vi "SLL DE DAQ Engine Main.vi"(8 "error in (no error)":errorcluster) -> (0 "error out":errorcluster)   [LabVIEW 2013]
uses:
  Controls/SLL DE DAQ Parameters LV2Global Options.ctl
  Controls/SLL DE DAQ Global Options.ctl
  Controls/SLL DE DI Global Options.ctl
  Controls/SLL DE AI Global Options.ctl
  Controls/SLL DE DO Global Options.ctl
  Controls/SLL DE AO Global Options.ctl
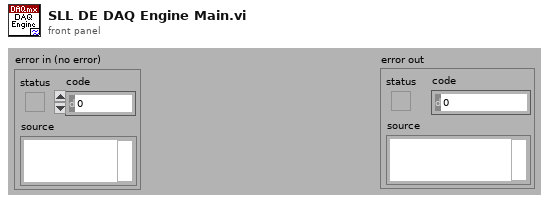
[diagram p1: front panel]
types:
  T1 = typedef "SLL DE DAQ Global Options.ctl" = enum16{"Init", "Write 1", "Read 1", "Write Array", "Read Array", "Clear"}
  T2 = typedef "SLL DE DAQ Parameters LV2Global Options.ctl" = enum16{"Read", "Write"}
  T3 = typedef "SLL DE DAQ Engine Parameters.ctl" = cluster{"Enable Engines":cluster{"AI Enable":bool, "AO Enable":bool, "DI Enable":bool, "DO Enable":bool}, "DAQ Control Type":cluster{"Analog Input":enum16{"Finite", "Continuous", "Driver"}, "Analog Output":enum16{"Finite", "Continuous", "Driver"}, "Digital Input":enum16{"Finite", "Continuous", "Driver"}, "Digital Output":enum16{"Finite", "Continuous", "Driver"}}, "DAQ Parameters":cluster{"AI Sampling Rate (Samples/Sec)":dbl, "MvgAVG Window Size (# of Points)":i32, "Enable Filter":bool, "Enable MvgAVG":bool, "Circular Buffer Size (Sec)":dbl, "AO Sampling Rate (Samples/Sec)":dbl, "Graph Update Rate (Samples/Sec)":dbl, "File Logging Rate (Samples/Sec)":i32}, "AO Safe Values":cluster{"Analog Outputs Name":T4, "Analog Outputs Safe Value":dbl}[], "DO Safe Values":cluster{"Digital Outputs Name":T5, "Digital Outputs Safe Value":bool}[], "DO Interconnected Lines":cluster{"First DO Line":string, "Second DO Line":string}[], "AI Channels Unit":cluster{"Channel Name":T6, "Channel Type":T7}[], "Units Information":cluster{"Channel Type":T7, "Unit Text":string, "Maximum":dbl, "Minmum":dbl, "Increments":dbl}[]}
  T4 = typedef "SLL DE List of Analog Outputs.ctl" = enum16{"None"}
  T5 = typedef "SLL DE List of Digital Outputs.ctl" = enum16{"STATION1_START TEST", "STATION1_STOP TEST", "STATION1_LIGHT1", "STATION1_LIGHT2", "STATION1_LIGHT3", "STATION1_SELECT_TEST", "STATION2_START TEST", "STATION2_STOP TEST", "STATION2_LIGHT1", "STATION2_LIGHT2", "STATION2_LIGHT3", "STATION2_SELECT_TEST", "STATION3_START TEST", "STATION3_STOP TEST", "STATION3_LIGHT1", "STATION3_LIGHT2", "STATION3_LIGHT3", "STATION3_SELECT_TEST", "STATION4_START TEST", "STATION4_STOP TEST", "STATION4_LIGHT1", "STATION4_LIGHT2", "STATION4_LIGHT3", "STATION4_SELECT_TEST"}
  T6 = typedef "SLL DE List of Analog Inputs.ctl" = enum16{"None"}
  T7 = typedef "SLL DE List of AI Channel Type.ctl" = enum16{"Pressure", "Flow", "Temperature", "Time Scale", "Voltage", "Current", "Frequency", "Sound", "Speed", "Torque", "Distance", "Channel Type 1", "Channel Type 2", "Channel Type 3"}
  T8 = typedef "SLL DE DI Global Options.ctl" = enum16{"Init", "Write Line", "Write Array", "Read Line", "Read Array", "Read Full Status", "Write Full Status"}
  T9 = typedef "SLL DE AO Global Options.ctl" = enum16{"Init", "Write Line", "Write Array", "Read Line", "Read Array", "Read Full Status", "Restart AO", "Send to Safe Mode", "Stop AO"}
  T10 = typedef "SLL DE DO Global Options.ctl" = enum16{"Init", "Write Line", "Write Array", "Write Full Status", "Read Line", "Read Array", "Read Full Status", "Restart DO", "Send to Safe Mode", "Stop DO"}
  T11 = typedef "SLL DE AI Global Options.ctl" = enum16{"Init", "Write Line", "Write Array", "Read Line", "Read Array", "Read Full Status", "Write Full Status"}
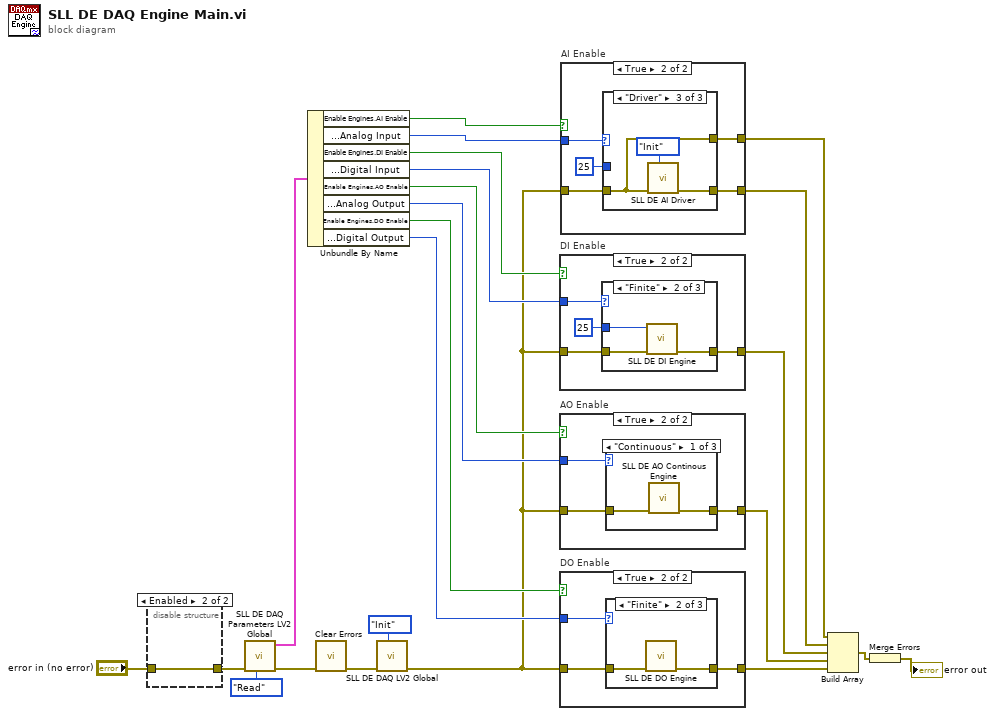
[diagram p0: block diagram]
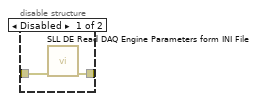
[diagram p2: hidden frame]
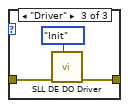
[diagram p5: hidden frame]
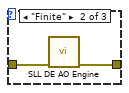
[diagram p7: hidden frame]
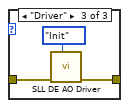
[diagram p8: hidden frame]
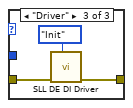
[diagram p11: hidden frame]
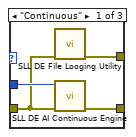
[diagram p13: hidden frame]
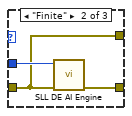
[diagram p14: hidden frame]
diagram:
  n1 = disable-structure shown="Enabled" {
    disable-tunnel: "error in (no error)" -> [w25 w26]
    disable-tunnel: [w24 w26] -> w9
    frame Disabled {
      n2 = call "SLL DE Read DAQ Engine Parameters form INI File.vi"("error in (no error)"=w25) -> ("error out"=w24:errorcluster)  [unwired: 10 out]
    }
    frame Enabled {
    }
  }
  n3 = call "SLL DE DAQ Parameters LV2 Global.vi"("Option"=SLL_DE_DAQ_Parameters_LV2Global_Options."Read", "Error in (no error)"=w9) -> ("Error out"=w8:errorcluster, "Global Info"=w7:T3)  [unwired: 1 in, 7 out]
  n4 = Unbundle By Name(w7) -> ("Enable Engines.AI Enable"=w4:bool, "DAQ Control Type.Analog Input"=w3:enum16{"Finite", "Continuous", "Driver"}, "Enable Engines.DI Enable"=w17:bool, "DAQ Control Type.Digital Input"=w18:enum16{"Finite", "Continuous", "Driver"}, "Enable Engines.AO Enable"=w15:bool, "DAQ Control Type.Analog Output"=w14:enum16{"Finite", "Continuous", "Driver"}, "Enable Engines.DO Enable"=w12:bool, "DAQ Control Type.Digital Output"=w11:enum16{"Finite", "Continuous", "Driver"})
  n5 = call <vilib>:"Clear Errors.vi"("error in (no error)"=w8) -> ("error out"=w6:errorcluster)  [unwired: 6 out]
  n6 = call "SLL DE DAQ LV2 Global.vi"("Option"=SLL_DE_DAQ_Global_Options."Init", "error in (no error)"=w6) -> ("error out"=w2:errorcluster)  [unwired: 4 in, 5 out]
  n7 = case "DI Enable" shown="True" w17 {
    tunnel: w2 -> [w27 w31]
    tunnel: [w27 w30] -> w19
    tunnel: w18 -> [_ w28]
    frame False {
    }
    frame True {
      n8 = case shown="\"Finite\"" w28 {
        tunnel: [w32 w34 w37] -> w30
        tunnel: u32 25 ("Delay (ms)") -> [_ w33 _]
        tunnel: w31 -> [w32 w35 w38]
        frame "Continuous" {
          # "Not\nApplicable"
        }
        frame "Finite" {
          n9 = call "SLL DE DI Engine.vi"("error in (no error)"=w35, "Delay (ms)"=w33) -> ("error out"=w34:errorcluster)  [unwired: 9 out]
        }
        frame "Driver" {
          n10 = call "SLL DE DI Driver.vi"("DI Driver Option"=SLL_DE_DI_Global_Options."Init", "error in (no error)"=w38) -> ("error out"=w37:errorcluster)  [unwired: 2 in, 7 out]
        }
      }
    }
  }
  n11 = case "AO Enable" shown="True" w15 {
    tunnel: w2 -> [w39 w42]
    tunnel: [w39 w41] -> w16
    tunnel: w14 -> [_ w40]
    frame False {
    }
    frame True {
      n12 = case shown="\"Continuous\"" w40 {
        tunnel: [w43 w45 w48] -> w41
        tunnel: w42 -> [w44 w46 w49]
        frame "Continuous" {
          n13 = call "SLL DE AO Continous Engine.vi"("error in (no error)"=w44) -> ("error out"=w43:errorcluster)  [unwired: 10 in]
        }
        frame "Finite" {
          n14 = call "SLL DE AO Engine.vi"("error in (no error)"=w46) -> ("error out"=w45:errorcluster)  [unwired: 1 in, 9 out]
        }
        frame "Driver" {
          n15 = call "SLL DE AO Driver.vi"("AO Driver Option"=SLL_DE_AO_Global_Options."Init", "error in (no error)"=w49) -> ("error out"=w48:errorcluster)  [unwired: 4 in, 5 out]
        }
      }
    }
  }
  n16 = case "DO Enable" shown="True" w12 {
    tunnel: w2 -> [w50 w53]
    tunnel: [w50 w52] -> w13
    tunnel: w11 -> [_ w51]
    frame False {
    }
    frame True {
      n17 = case shown="\"Finite\"" w51 {
        tunnel: [w54 w55 w57] -> w52
        tunnel: w53 -> [w54 w56 w58]
        frame "Continuous" {
          # "Not\nApplicable"
        }
        frame "Finite" {
          n18 = call "SLL DE DO Engine.vi"("error in (no error)"=w56) -> ("error out"=w55:errorcluster)  [unwired: 1 in, 9 out]
        }
        frame "Driver" {
          n19 = call "SLL DE DO Driver.vi"("DO Driver Option"=SLL_DE_DO_Global_Options."Init", "error in (no error)"=w58) -> ("error out"=w57:errorcluster)  [unwired: 4 in, 5 out]
        }
      }
    }
  }
  n20 = case "AI Enable" shown="True" w4 {
    tunnel: [w60 w65] -> w22
    tunnel: w2 -> [w60 w63]
    tunnel: w3 -> [_ w62]
    tunnel: [w60 w61] -> w1
    frame False {
    }
    frame True {
      n21 = case shown="\"Driver\"" w62 {
        tunnel: [w69 w70 w74] -> w65
        tunnel: u32 25 ("Delay (ms)") -> [w68 w72 _]
        tunnel: w63 -> [w66 w71 w73]
        tunnel: [w67 w71 w73] -> w61
        frame "Continuous" {
          n22 = call "SLL DE File Looging Utility.vi"("error in (no error)"=w66) -> ("error out"=w67:errorcluster)  [unwired: 10 in]
          n23 = call "SLL DE AI Continuous Engine.vi"("error in (no error)"=w66, "Delay (ms)"=w68) -> ("error out"=w69:errorcluster)  [unwired: 9 out]
        }
        frame "Finite" {
          n24 = call "SLL DE AI Engine.vi"("error in (no error)"=w71, "Delay (ms)"=w72) -> ("error out"=w70:errorcluster)  [unwired: 9 out]
        }
        frame "Driver" {
          n25 = call "SLL DE AI Driver.vi"("AI Driver Option"=SLL_DE_AI_Global_Options."Init", "error in (no error)"=w73) -> ("error out"=w74:errorcluster)  [unwired: 2 in, 7 out]
        }
      }
    }
  }
  n26 = Build Array(w1, w22, w19, w16, w13) -> (w21:errorcluster[])
  n27 = Merge Errors(w21) -> (→"error out":errorcluster)
